vi "Mark_BE_Peak.vi"(4 "Output Type":enum16{"Time", "Percentage", "Index"}(ring), 5 "End Time":dbl, 6 "HalfWidth":i32, 7 "Start Time":dbl, 8 "error in (no error)":errorcluster, 9 "Input":dbl[](array[numeric]), 10 "Time":dbl[](array[numeric]), 11 "CarexData In":refnum<class "ExpData.lvclass">) -> (0 "error out":errorcluster, 1 "End":dbl[](array[numeric]) format="%.2f", 2 "Begin":dbl[](array[numeric]) format="%.2f", 3 "CarexData Out":refnum<class "ExpData.lvclass">)   [LabVIEW 2016, in "ExpData.lvclass"]
uses:
  ExpData.lvclass
  ExpData.lvclass/ExpData.ctl
  <userlib>/_OpenG.lib/array/array.llb/Conditional Auto-Indexing Tunnel (I32)__ogtk.vi
  <userlib>/_OpenG.lib/array/array.llb/Index 1D Array Elements (DBL)__ogtk.vi
  <vilib>/AuZn/auzn custom VIs/AuZnCustomVI.lvlib
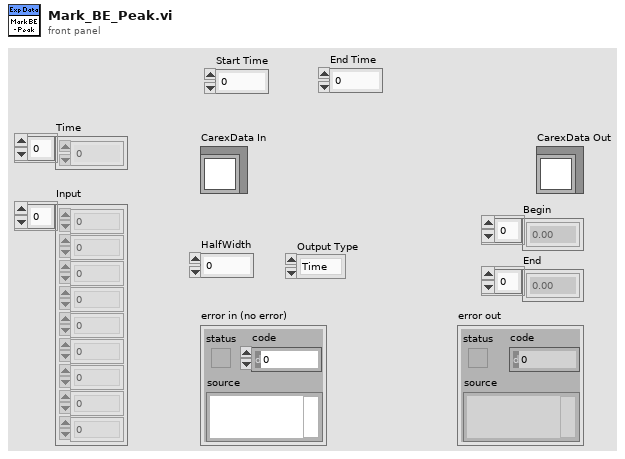
[diagram p1: front panel]
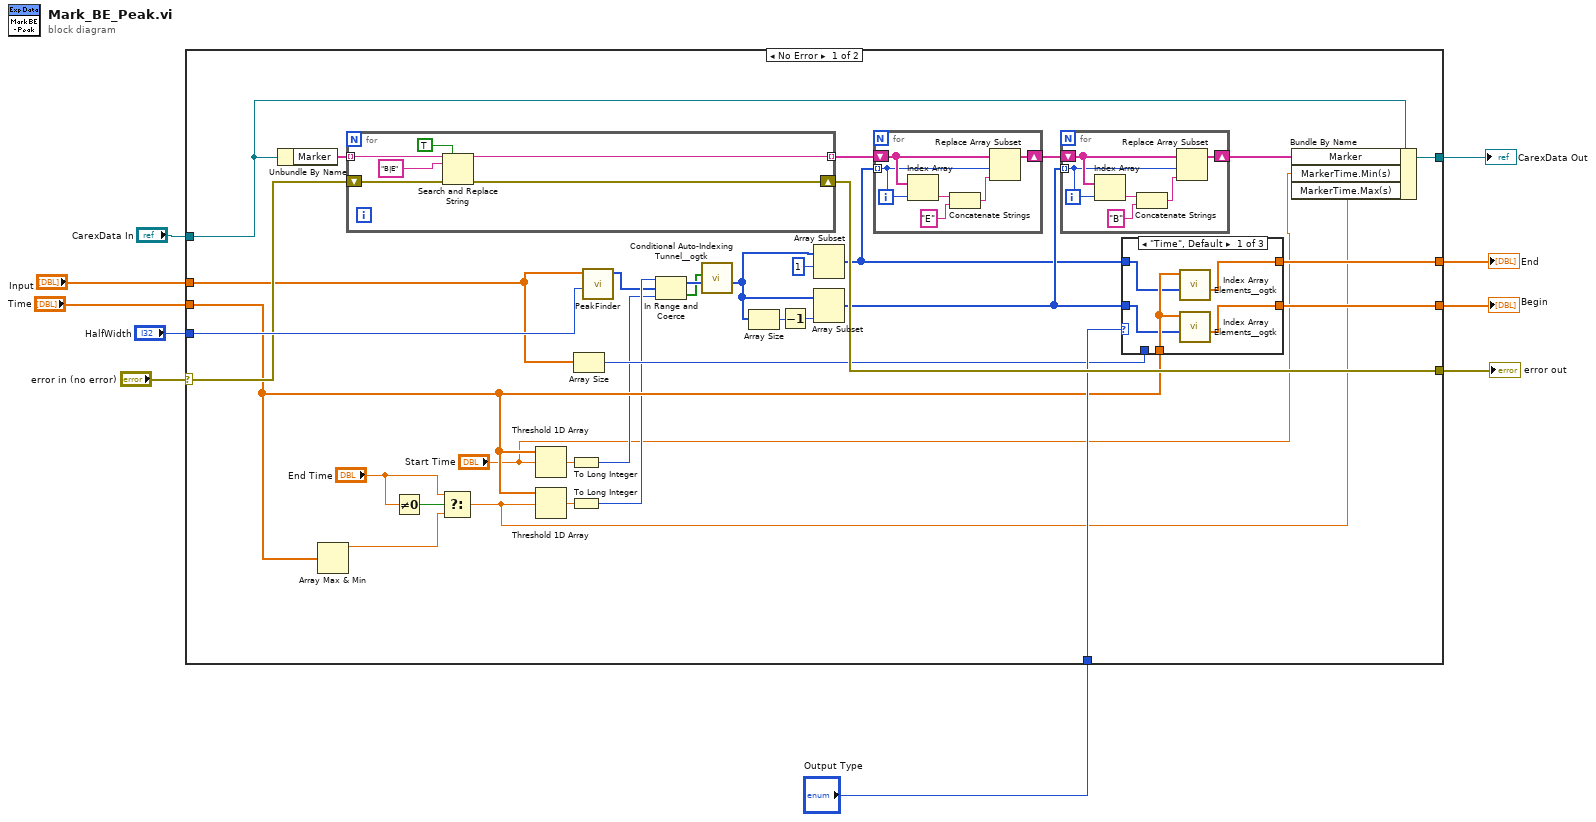
[diagram p0: block diagram]
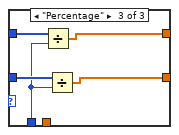
[diagram p3: hidden frame]
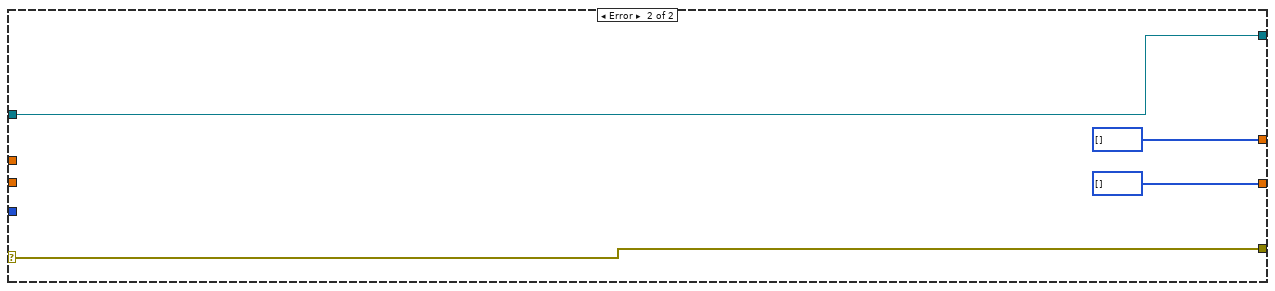
[diagram p4: hidden frame]
diagram:
  n1 = case shown="No Error" "error in (no error)" {
    selector: "error in (no error)" -> [w26 w77]
    tunnel: [w37 w77] -> w10
    tunnel: "CarexData In" -> [w27 w74]
    tunnel: "HalfWidth" -> [w43 _]
    tunnel: [w32 i32[] []] -> w6
    tunnel: [w30 i32[] []] -> w5
    tunnel: [w35 w74] -> w4
    tunnel: "Output Type" -> [w29 _]
    tunnel: "Time" -> [w19 _]
    tunnel: "Input" -> [w25 _]
    frame No Error {
      n2 = Unbundle By Name(w27) -> ("Marker"=w34:string[])
      n3 = Array Max & Min(array=w19) -> (max value=w22:dbl)  [unwired: 3 out]
      n4 = for {
        tunnel: w34 -> [w61] mode=indexing
        tunnel: [w59] -> w38 mode=indexing
        shift-right: [w56] -> w37
        shift-left: w26 -> [w57]
        n5 = Search and Replace String(replace all?=TRUE ("replace all? (F)"), input string=w61, search string="B|E", error in=w57) -> (result string=w59:string, error out=w56:errorcluster)  [unwired: 4 in, 2 out]
      }
      n6 = Not Equal To 0?(x="End Time") -> (x != 0?=w23:bool)
      n7 = Select(t="End Time", s=w23, f=w22) -> (s? t:f=w12:dbl)
      n8 = Threshold 1D Array(2:"Start Time", 3:w19) -> (0:w20:dbl)  [unwired: 1 in]
      n9 = Threshold 1D Array(2:w12, 3:w19) -> (0:w21:dbl)  [unwired: 1 in]
      n10 = To Long Integer(number=w20) -> (32bit integer=w17:i32)
      n11 = To Long Integer(number=w21) -> (32bit integer=w18:i32)
      n12 = Array Size(array=w25) -> (size(s)=w28:i32)
      n13 = call <vilib>:"PeakFinder.vi"("HalfWidth(10)"=w43, "Input"=w25) -> ("PeakPos"=w11:i32[])  [unwired: 4 in, 3 out]
      n14 = In Range and Coerce(upper limit=w18, x=w11, lower limit=w17) -> (coerced(x)=w16:i32[], In Range?=w15:bool[])
      n15 = call-poly <userlib>:"Conditional Auto-Indexing Tunnel__ogtk.vi"("Array in"=w16, "Elements to keep"=w15) -> ("Filtered Array out"=w14:i32[])  [unwired: 5 in]
      n16 = Array Size(array=w14) -> (size(s)=w42:i32)
      n17 = Decrement(x=w42) -> (x-1=w41:i32)
      n18 = Array Subset(array=w14, index=1) -> (w31:i32[])  [unwired: 1 in]
      n19 = Array Subset(array=w14, length=w41) -> (w33:i32[])  [unwired: 1 in]
      n20 = for {
        tunnel: w31 -> [w71] mode=indexing
        shift-right: [w73] -> w39
        shift-left: w38 -> [w72]
        n21 = Index Array(array=w72, index=w71) -> (element=w69:string)
        n22 = Concatenate Strings(w69, "E" ("new element/subarray")) -> (w70:string)
        n23 = Replace Array Subset(array=w72, new element=w70, index=w71) -> (w73:string[])
      }
      n24 = for {
        tunnel: w33 -> [w65] mode=indexing
        shift-right: [w67] -> w36
        shift-left: w39 -> [w66]
        n25 = Index Array(array=w66, index=w65) -> (element=w63:string)
        n26 = Concatenate Strings(w63, "B" ("new element/subarray")) -> (w64:string)
        n27 = Replace Array Subset(array=w66, new element=w64, index=w65) -> (w67:string[])
      }
      n28 = case shown="\"Time\", Default" w29 {
        tunnel: w33 -> [w45 w50 w53]
        tunnel: [w44 w50 w51] -> w32
        tunnel: w31 -> [w47 w49 w55]
        tunnel: [w46 w49 w54] -> w30
        tunnel: w28 -> [_ _ w52]
        tunnel: w19 -> [w48 _ _]
        frame "Time", Default {
          n29 = call-poly <userlib>:"Index Array Elements__ogtk.vi"("indices"=w47, "array"=w48) -> ("elements"=w46:dbl[])  [unwired: 9 in]
          n30 = call-poly <userlib>:"Index Array Elements__ogtk.vi"("indices"=w45, "array"=w48) -> ("elements"=w44:dbl[])  [unwired: 9 in]
        }
        frame "Index" {
        }
        frame "Percentage" {
          n31 = Divide(x=w55, y=w52) -> (x/y=w54:dbl[])
          n32 = Divide(x=w53, y=w52) -> (x/y=w51:dbl[])
        }
      }
      n33 = Bundle By Name(cluster=w27, "Marker"=w36, "MarkerTime.Min(s)"="Start Time", "MarkerTime.Max(s)"=w12) -> (w35:refnum<class "ExpData.lvclass">)
    }
    frame Error {
    }
  }
  "CarexData Out" <- w4
  "error out" <- w10
  "Begin" <- w6
  "End" <- w5
